vi "Communication - Handle (FGV).vi"(7 "Action":T1, 8 "error in (no error)":errorcluster, 9 "S/N":string, 10 "S/N Array":string[](array[string]), 11 "Handle":u32[](array[numeric])) -> (0 "error out":errorcluster, 2 "Handle":u32, 3 "Handle Out":u32[](array[numeric]))   [LabVIEW 2019]
uses:
  Controls/FGV States.ctl
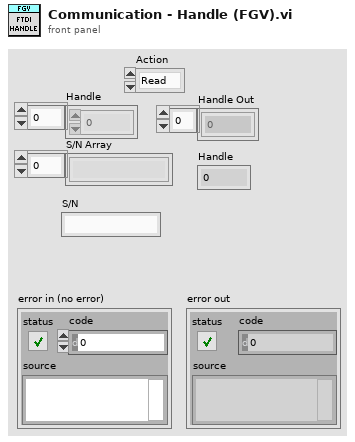
[diagram p1: front panel]
types:
  T1 = typedef "FGV States.ctl" = enum16{"Read", "Write"}
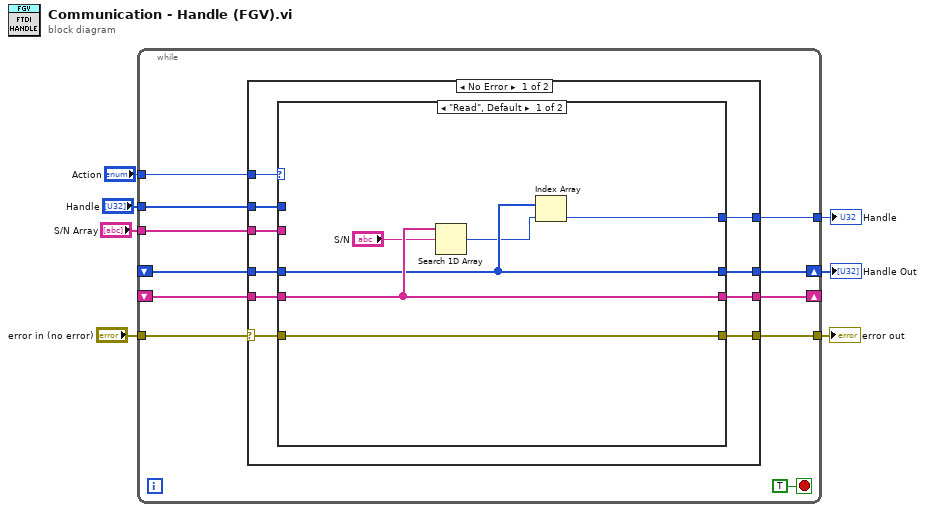
[diagram p0: block diagram]
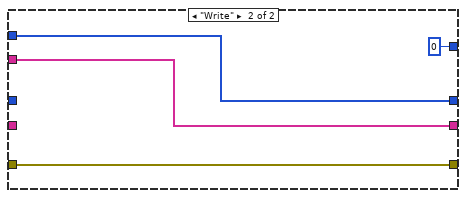
[diagram p2: hidden frame]
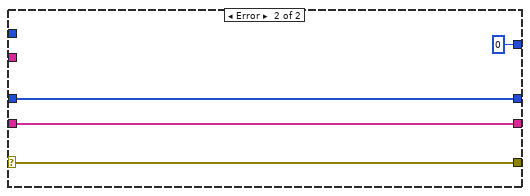
[diagram p3: hidden frame]
diagram:
  n1 = while {
    tunnel: "Action" -> [w18]
    tunnel: "Handle" -> [w16]
    shift-right: [w17] -> w3
    shift-left: _ -> [w15]
    tunnel: "error in (no error)" -> [w13]
    tunnel: [w12] -> w4
    tunnel: "S/N Array" -> [w10]
    shift-right: [w11] -> _
    shift-left: _ -> [w9]
    tunnel: [w8] -> w1
    stop <- TRUE stop-if-true
    n2 = case shown="No Error" w13 {
      selector: w13 -> [w23 w41]
      tunnel: w18 -> [w28 _]
      tunnel: [w27 w42] -> w17
      tunnel: w16 -> [w26 _]
      tunnel: w15 -> [w25 w42]
      tunnel: [w24 w41] -> w12
      tunnel: [w22 w40] -> w11
      tunnel: w10 -> [w21 _]
      tunnel: w9 -> [w20 w40]
      tunnel: [w19 u32 0 ("Handle 2")] -> w8
      frame No Error {
        n3 = case shown="\"Read\", Default" w28 {
          tunnel: [w31 w38] -> w27
          tunnel: w26 -> [_ w38]
          tunnel: w25 -> [w31 _]
          tunnel: [w34 w37] -> w24
          tunnel: w23 -> [w34 w37]
          tunnel: [w33 w36] -> w22
          tunnel: w21 -> [_ w36]
          tunnel: w20 -> [w33 _]
          tunnel: [w29 u32 0 ("Handle 2")] -> w19
          frame "Read", Default {
            n4 = Search 1D Array(1D array=w33, element="S/N") -> (index of element=w30:i32)  [unwired: 1 in]
            n5 = Index Array(array=w31, index=w30) -> (element=w29:u32)
          }
          frame "Write" {
          }
        }
      }
      frame Error {
      }
    }
  }
  "error out" <- w4
  "Handle Out" <- w3
  "Handle" <- w1
